vi "TE - Read error code.vi"(2 "error in":errorcluster, 3 "Address / Port":i16=1 min=1 max=31 step=1) -> (0 "error out":errorcluster, 1 "Read error code":dbl format="%.2f")   [LabVIEW 2014]
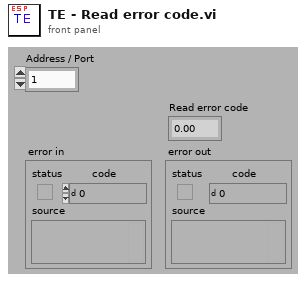
[diagram p1: front panel]
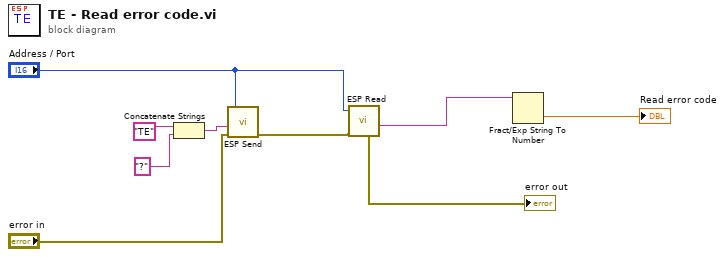
[diagram p0: block diagram]
diagram:
  n1 = Concatenate Strings("TE" ("Substring"), "?" ("Substring")) -> (w8:string)
  n2 = call "ESP Send.vi"("Address / Port"="Address / Port", "Command String"=w8, "error in"="error in") -> ("error out"=w3:errorcluster)  [unwired: 5 in]
  n3 = call "ESP Read.vi"("Address / Port"="Address / Port", "error in"=w3) -> ("error out"=→"error out":errorcluster, "Response String"=w5:string)  [unwired: 5 in]
  n4 = Fract/Exp String To Number(string=w5) -> (number=→"Read error code":dbl)  [unwired: 3 in, 1 out]
